vi "Read Typedefs.vi"(8 "error in (no error)":errorcluster, 11 "Kobe Bryant in":refnum<class "Kobe Bryant.lvclass">) -> (0 "error out":errorcluster, 2 "Cluster":T1, 3 "Kobe Bryant out":refnum<class "Kobe Bryant.lvclass">)   [LabVIEW 2019, in "Kobe Bryant.lvclass"]
uses:
  Kobe Bryant.lvclass
  KobeData1.ctl
  KobeData2.ctl
  KobeEnum.ctl
  Kobe Bryant.lvclass/Kobe Bryant.ctl
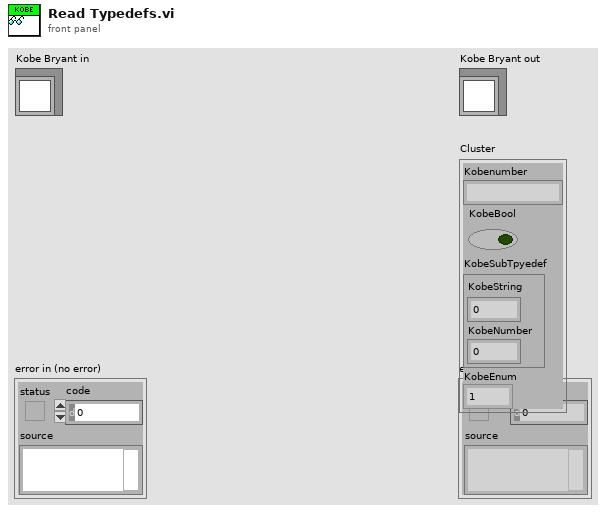
[diagram p1: front panel]
types:
  T1 = typedef "Kobe Bryant.lvclass/KobeData1.ctl" = cluster{"Kobenumber":string, "KobeBool":bool, "KobeSubTpyedef":T2, "KobeEnum":T3}
  T2 = typedef "Kobe Bryant.lvclass/KobeData2.ctl" = cluster{"KobeString":dbl, "KobeNumber":dbl}
  T3 = typedef "Kobe Bryant.lvclass/KobeEnum.ctl" = enum16{"1", "2", "3", "4", "5"}
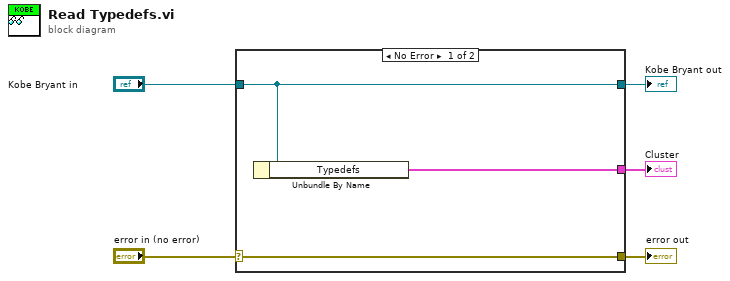
[diagram p0: block diagram]
diagram:
  n1 = case shown="No Error" "error in (no error)" {
    selector: "error in (no error)" -> [w8 w9]
    tunnel: [w8 w9] -> w4
    tunnel: [w7 w10] -> w2
    tunnel: "Kobe Bryant in" -> [w7 w10]
    tunnel: [w6 _] -> w1
    frame No Error {
      n2 = Unbundle By Name(w7) -> ("Typedefs"=w6:T1)
    }
    frame Error {
    }
  }
  "error out" <- w4
  "Kobe Bryant out" <- w2
  "Cluster" <- w1
